vi "SetPosHardware.vi"(6 "RealMove":dbl, 7 "SingleMove?":bool, 8 "error in (no error)":errorcluster, 9 "Axis 1":string, 10 "FirstMove":dbl, 11 "XPS-RLD in":refnum<class "XPS-RLD.lvclass">) -> (0 "error out":errorcluster, 3 "XPS-RLD out":refnum<class "XPS-RLD.lvclass">)   [LabVIEW 2020, in "XPS-RLD.lvclass"]
uses:
  XPS-RLD/XPS-RLD.lvclass
  XPS-RLD/XPS-RLD.lvclass/XPS-RLD.ctl
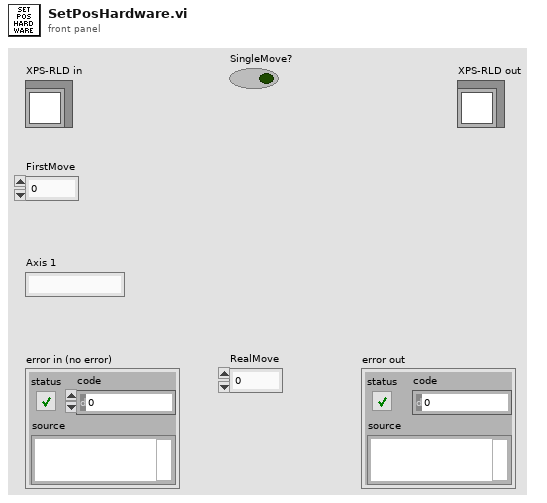
[diagram p1: front panel]
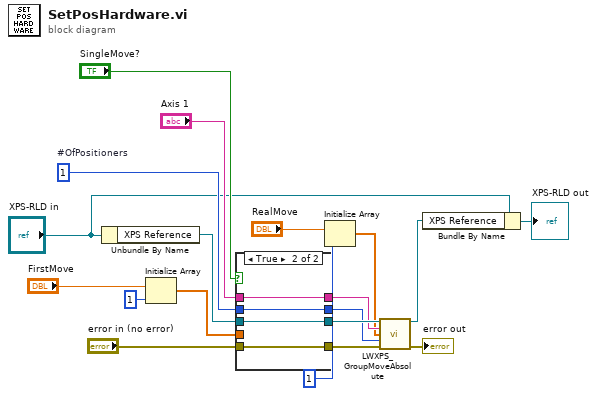
[diagram p0: block diagram]
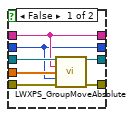
[diagram p2: hidden frame]
diagram:
  w6 = 1  # #OfPositioners
  n1 = Unbundle By Name("XPS-RLD in") -> ("XPS Reference"=w19:refnum<k24>)
  n2 = Initialize Array("FirstMove", 1 ("dimension size")) -> (w7:dbl[])
  n3 = case shown="True" "SingleMove?" {
    tunnel: "Axis 1" -> [w21 w29]
    tunnel: "error in (no error)" -> [w24 w30]
    tunnel: [w23 w30] -> w15
    tunnel: w19 -> [w26 w28]
    tunnel: [w21 w29] -> w11
    tunnel: [w25 w28] -> w12
    tunnel: w7 -> [w22 _]
    tunnel: w6 -> [w20 w27]
    tunnel: [w20 w27] -> w5
    frame False {
      n4 = call "LWXPS_GroupMoveAbsolute.vi"("CommandInterfaceXPS.XPS"=w26, "Group Name"=w21, "Target Position IN"=w22, "Number of Positioners"=w20, "LabVIEW error IN"=w24) -> ("CommandInterfaceXPS.XPS"=w25:refnum<k24>, "LabVIEW error OUT"=w23:errorcluster)  [unwired: 6 in, 3 out]
    }
    frame True {
    }
  }
  n5 = Initialize Array("RealMove", 1 ("dimension size")) -> (w9:dbl[])
  n6 = call "LWXPS_GroupMoveAbsolute.vi"("CommandInterfaceXPS.XPS"=w12, "Group Name"=w11, "Target Position IN"=w9, "Number of Positioners"=w5, "LabVIEW error IN"=w15) -> ("CommandInterfaceXPS.XPS"=w13:refnum<k24>, "LabVIEW error OUT"=→"error out":errorcluster)  [unwired: 6 in, 3 out]
  n7 = Bundle By Name(cluster="XPS-RLD in", "XPS Reference"=w13) -> (→"XPS-RLD out":refnum<class "XPS-RLD.lvclass">)
